vi "AdaptToInputs.vi"(3 "Term Types":T1[](array[typedef]), 4 "XRef":refnum<vi>, 5 "State In":T4={"Input Type"=variant(path path ""), "Terminals"=[]}) -> (0 "Reply":string[](array[string]), 2 "State Out":T4={"Input Type"=variant(path path ""), "Terminals"=[]})   [LabVIEW 2015, in "Await.xnode"]
doc: "This ability VI is called by LabVIEW during type propagation so that your XNode may adapt itself to new input types. Term Types is an array of pairs of current Term IDs and the type descriptors corresponding to them. The type descriptors are taken from the signal connected to the terminal. Unwired terminals are not included in the array. Use Reply to inform LabVIEW of any actions it needs to take.\n\nDefault behavior: None.\n\nThis ability does not provide UI and OS messages are not handled."
uses:
  Await.xnode
  State.ctl
  <vilib>/XNodeSupport/XNodeTermTypeIDPair.ctl
  <vilib>/XNodeSupport/XNodeType.ctl
  <vilib>/XNodeSupport/XNodeString.ctl
  <vilib>/Erdos Miller/LV-Scripting/LV-Scripting.lvlib
  <vilib>/Utility/Data Type/NI_Data Type.lvlib
  <vilib>/XNodeSupport/NI_XNodeSupport.lvlib
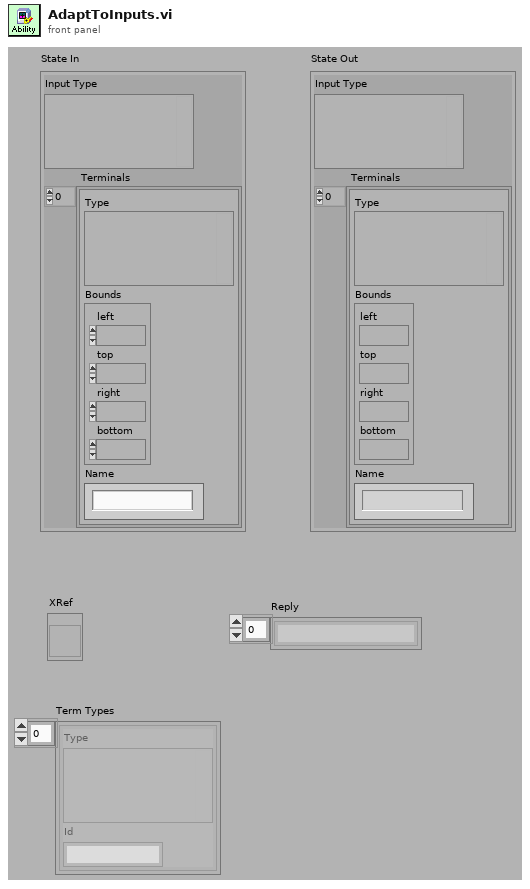
[diagram p1: front panel]
types:
  T1 = typedef "NI_XNodeSupport.lvlib/XNodeTermTypeIDPair.ctl" = cluster{"Type":T2, "Id":T3}
  T2 = typedef "NI_XNodeSupport.lvlib/XNodeType.ctl" = variant
  T3 = typedef "NI_XNodeSupport.lvlib/XNodeString.ctl" = string
  T4 = typedef "Await.xnode/State.ctl" = cluster{"Input Type":variant, "Terminals":cluster{"Type":variant, "Bounds":cluster{"left":i16, "top":i16, "right":i16, "bottom":i16}, "Name":string}[]}
  T5 = cluster{"Connector":i32, "Rects":cluster{"left":i16, "top":i16, "right":i16, "bottom":i16}[]}[]
  T6 = typedef "NI_Data Type.lvlib/VI Info.ctl" = cluster{"Connector Pane Pattern":i16, "Connector Pane Rotation":i16, "Flags":u32[], "Modification Date":timestamp, "Asynchronous":bool, "Non-Function":bool, "Subroutine":bool, "SubSystem":bool}
  T7 = cluster{"Connector":i32, "Rects":cluster{"left":i16, "top":i16, "right":i16, "bottom":i16}[]}
  T8 = cluster{"left":i16, "top":i16, "right":i16, "bottom":i16}[]
  T9 = cluster{"Variant":variant, "Rect":cluster{"left":i16, "top":i16, "right":i16, "bottom":i16}, "Name":string}
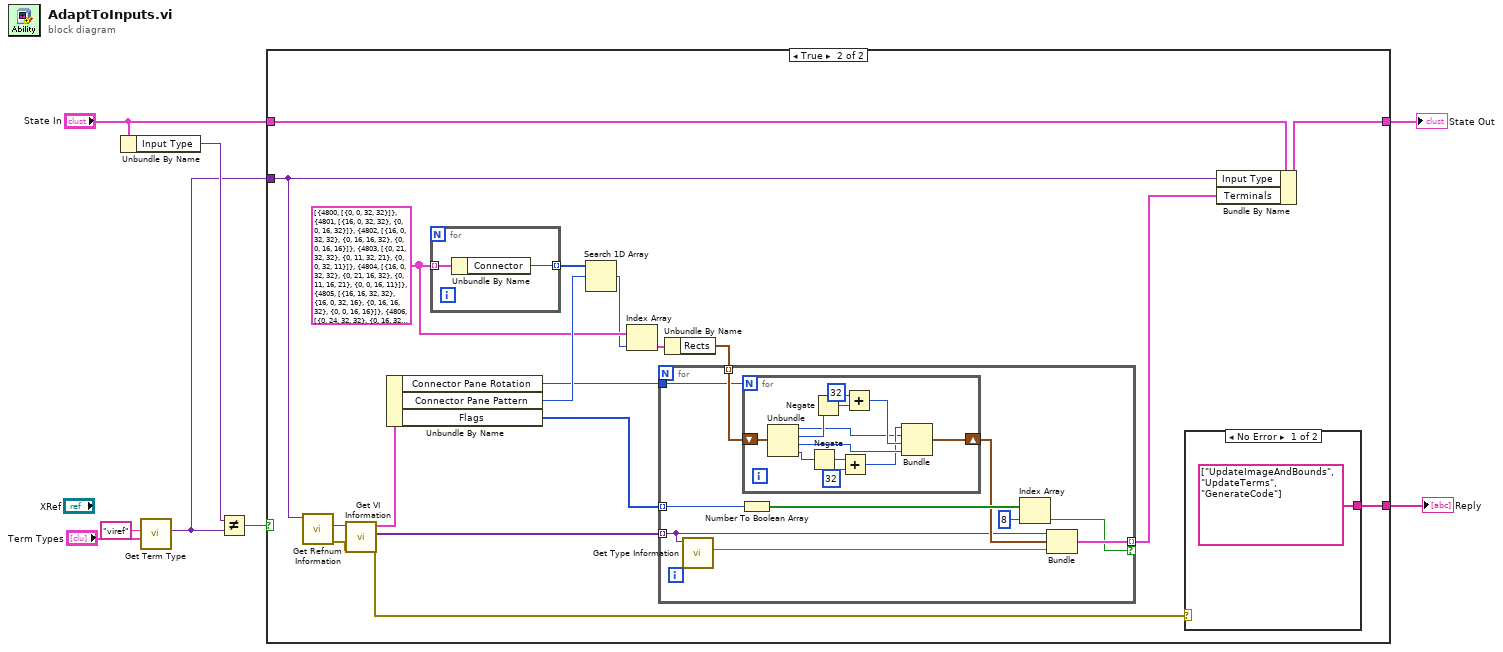
[diagram p0: block diagram]
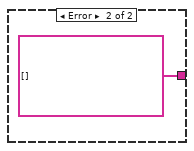
[diagram p3: hidden frame]
diagram:
  n1 = Unbundle By Name("State In") -> ("Input Type"=w6:variant)
  n2 = call <vilib>:"Get Term Type.vi"("Term Types"="Term Types", "ID"="viref") -> ("Type"=w2:variant)  [unwired: 9 in]
  n3 = Not Equal?(x=w6, y=w2) -> (x != y?=w5:bool)
  n4 = case shown="True" w5 {
    tunnel: [w9 w26] -> w4
    tunnel: "State In" -> [w9 w27]
    tunnel: w2 -> [_ w25]
    tunnel: [_ w13] -> w1
    frame False {
    }
    frame True {
      w18 = T5 [{"Connector"=4800, "Rects"=[{"left"=0, "top"=0, "right"=32, "bottom"=32}]}, {"Connector"=4801, "Rects"=[{"left"=16, "top"=0, "right"=32, "bottom"=32}, {"left"=0, "top"=0, "right"=16, "bottom"=32}]}, {"Connector"=4802, "Rects"=[{"left"=16, "top"=0, "right"=32, "bottom"=32}, {"left"=0, "top"=16, "right"=16, "bottom"=32}, {"left"=0, "top"=0, "right"=16, "bottom"=16}]}, {"Connector"=4803, "Rects"=[{"left"=0, "top"=21, "right"=32, "bottom"=32}, {"left"=0, "top"=11, "right"=32, "bottom"=21}, {"left"=0, "top"=0, "right"=32, "bottom"=11}]}, {"Connector"=4804, "Rects"=[{"left"=16, "top"=0, "right"=32, "bottom"=32}, {"left"=0, "top"=21, "right"=16, "bottom"=32}, {"left"=0, "top"=11, "right"=16, "bottom"=21}, {"left"=0, "top"=0, "right"=16, "bottom"=11}]}, {"Connector"=4805, "Rects"=[{"left"=16, "top"=16, "right"=32, "bottom"=32}, {"left"=16, "top"=0, "right"=32, "bottom"=16}, {"left"=0, "top"=16, "right"=16, "bottom"=32}, {"left"=0, "top"=0, "right"=16, "bottom"=16}]}, {"Connector"=4806, "Rects"=[{"left"=0, "top"=24, "right"=32, "bottom"=32}, {"left"=0, "top"=16, "right"=32, "bottom"=24}, {"left"=0, "top"=8, "right"=32, "bottom"=16}, {"left"=0, "top"=0, "right"=32, "bottom"=8}]}, {"Connector"=4807, "Rects"=[{"left"=16, "top"=16, "right"=32, "bottom"=32}, {"left"=16, "top"=0, "right"=32, "bottom"=16}, {"left"=0, "top"=21, "right"=16, "bottom"=32}, {"left"=0, "top"=11, "right"=16, "bottom"=21}, {"left"=0, "top"=0, "right"=16, "bottom"=11}]}, {"Connector"=4808, "Rects"=[{"left"=16, "top"=0, "right"=32, "bottom"=32}, {"left"=0, "top"=24, "right"=16, "bottom"=32}, {"left"=0, "top"=16, "right"=16, "bottom"=24}, {"left"=0, "top"=8, "right"=16, "bottom"=16}, {"left"=0, "top"=0, "right"=16, "bottom"=8}]}, {"Connector"=4809, "Rects"=[{"left"=16, "top"=16, "right"=32, "bottom"=32}, {"left"=16, "top"=0, "right"=32, "bottom"=16}, {"left"=0, "top"=24, "right"=16, "bottom"=32}, {"left"=0, "top"=16, "right"=16, "bottom"=24}, {"left"=0, "top"=8, "right"=16, "bottom"=16}, {"left"=0, "top"=0, "right"=16, "bottom"=8}]}, {"Connector"=4810, "Rects"=[{"left"=16, "top"=21, "right"=32, "bottom"=32}, {"left"=16, "top"=11, "right"=32, "bottom"=21}, {"left"=16, "top"=0, "right"=32, "bottom"=11}, {"left"=0, "top"=21, "right"=16, "bottom"=32}, {"left"=0, "top"=11, "right"=16, "bottom"=21}, {"left"=0, "top"=0, "right"=16, "bottom"=11}]}, {"Connector"=4811, "Rects"=[{"left"=16, "top"=21, "right"=32, "bottom"=32}, {"left"=16, "top"=11, "right"=32, "bottom"=21}, {"left"=16, "top"=0, "right"=32, "bottom"=11}, {"left"=0, "top"=24, "right"=16, "bottom"=32}, {"left"=0, "top"=16, "right"=16, "bottom"=24}, {"left"=0, "top"=8, "right"=16, "bottom"=16}, {"left"=0, "top"=0, "right"=16, "bottom"=8}]}, {"Connector"=4812, "Rects"=[{"left"=16, "top"=24, "right"=32, "bottom"=32}, {"left"=16, "top"=16, "right"=32, "bottom"=24}, {"left"=16, "top"=8, "right"=32, "bottom"=16}, {"left"=16, "top"=0, "right"=32, "bottom"=8}, {"left"=0, "top"=24, "right"=16, "bottom"=32}, {"left"=0, "top"=16, "right"=16, "bottom"=24}, {"left"=0, "top"=8, "right"=16, "bottom"=16}, {"left"=0, "top"=0, "right"=16, "bottom"=8}]}, {"Connector"=4813, "Rects"=[{"left"=16, "top"=24, "right"=32, "bottom"=32}, {"left"=16, "top"=16, "right"=32, "bottom"=24}, {"left"=16, "top"=8, "right"=32, "bottom"=16}, {"left"=16, "top"=0, "right"=32, "bottom"=8}, {"left"=8, "top"=0, "right"=16, "bottom"=32}, {"left"=0, "top"=24, "right"=8, "bottom"=32}, {"left"=0, "top"=16, "right"=8, "bottom"=24}, {"left"=0, "top"=8, "right"=8, "bottom"=16}, {"left"=0, "top"=0, "right"=8, "bottom"=8}]}, {"Connector"=4814, "Rects"=[{"left"=16, "top"=24, "right"=32, "bottom"=32}, {"left"=16, "top"=16, "right"=32, "bottom"=24}, {"left"=16, "top"=8, "right"=32, "bottom"=16}, {"left"=16, "top"=0, "right"=32, "bottom"=8}, {"left"=8, "top"=16, "right"=16, "bottom"=32}, {"left"=8, "top"=0, "right"=16, "bottom"=16}, {"left"=0, "top"=24, "right"=8, "bottom"=32}, {"left"=0, "top"=16, "right"=8, "bottom"=24}, {"left"=0, "top"=8, "right"=8, "bottom"=16}, {"left"=0, "top"=0, "right"=8, "bottom"=8}]}, {"Connector"=4815, "Rects"=[{"left"=24, "top"=24, "right"=32, "bottom"=32}, {"left"=24, "top"=16, "right"=32, "bottom"=24}, {"left"=24, "top"=8, "right"=32, "bottom"=16}, {"left"=24, "top"=0, "right"=32, "bottom"=8}, {"left"=16, "top"=16, "right"=24, "bottom"=32}, {"left"=16, "top"=0, "right"=24, "bottom"=16}, {"left"=8, "top"=16, "right"=16, "bottom"=32}, {"left"=8, "top"=0, "right"=16, "bottom"=16}, {"left"=0, "top"=24, "right"=8, "bottom"=32}, {"left"=0, "top"=16, "right"=8, "bottom"=24}, {"left"=0, "top"=8, "right"=8, "bottom"=16}, {"left"=0, "top"=0, "right"=8, "bottom"=8}]}, {"Connector"=4816, "Rects"=[{"left"=0, "top"=0, "right"=8, "bottom"=11}, {"left"=8, "top"=0, "right"=16, "bottom"=11}, {"left"=0, "top"=11, "right"=16, "bottom"=21}, {"left"=0, "top"=21, "right"=8, "bottom"=32}, {"left"=8, "top"=21, "right"=16, "bottom"=32}, {"left"=16, "top"=0, "right"=32, "bottom"=32}]}, {"Connector"=4817, "Rects"=[{"left"=0, "top"=0, "right"=8, "bottom"=11}, {"left"=8, "top"=0, "right"=16, "bottom"=11}, {"left"=0, "top"=11, "right"=16, "bottom"=21}, {"left"=0, "top"=21, "right"=8, "bottom"=32}, {"left"=8, "top"=21, "right"=16, "bottom"=32}, {"left"=16, "top"=0, "right"=32, "bottom"=16}, {"left"=16, "top"=16, "right"=32, "bottom"=32}]}, {"Connector"=4818, "Rects"=[{"left"=0, "top"=0, "right"=8, "bottom"=11}, {"left"=8, "top"=0, "right"=16, "bottom"=11}, {"left"=0, "top"=11, "right"=16, "bottom"=21}, {"left"=0, "top"=21, "right"=8, "bottom"=32}, {"left"=8, "top"=21, "right"=16, "bottom"=32}, {"left"=16, "top"=0, "right"=32, "bottom"=11}, {"left"=16, "top"=11, "right"=32, "bottom"=21}, {"left"=16, "top"=21, "right"=32, "bottom"=32}]}, {"Connector"=4819, "Rects"=[{"left"=0, "top"=0, "right"=8, "bottom"=11}, {"left"=8, "top"=0, "right"=16, "bottom"=11}, {"left"=0, "top"=11, "right"=16, "bottom"=21}, {"left"=0, "top"=21, "right"=8, "bottom"=32}, {"left"=8, "top"=21, "right"=16, "bottom"=32}, {"left"=16, "top"=0, "right"=32, "bottom"=8}, {"left"=16, "top"=8, "right"=32, "bottom"=16}, {"left"=16, "top"=16, "right"=32, "bottom"=24}, {"left"=16, "top"=24, "right"=32, "bottom"=32}]}, {"Connector"=4820, "Rects"=[{"left"=0, "top"=0, "right"=8, "bottom"=11}, {"left"=8, "top"=0, "right"=16, "bottom"=11}, {"left"=0, "top"=11, "right"=16, "bottom"=21}, {"left"=0, "top"=21, "right"=8, "bottom"=32}, {"left"=8, "top"=21, "right"=16, "bottom"=32}, {"left"=16, "top"=0, "right"=24, "bottom"=11}, {"left"=24, "top"=0, "right"=32, "bottom"=11}, {"left"=16, "top"=11, "right"=32, "bottom"=21}, {"left"=16, "top"=21, "right"=24, "bottom"=32}, {"left"=24, "top"=21, "right"=32, "bottom"=32}]}, {"Connector"=4821, "Rects"=[{"left"=0, "top"=0, "right"=8, "bottom"=11}, {"left"=8, "top"=0, "right"=16, "bottom"=11}, {"left"=0, "top"=11, "right"=16, "bottom"=21}, {"left"=0, "top"=21, "right"=8, "bottom"=32}, {"left"=8, "top"=21, "right"=16, "bottom"=32}, {"left"=16, "top"=0, "right"=24, "bottom"=16}, {"left"=24, "top"=0, "right"=32, "bottom"=8}, {"left"=24, "top"=8, "right"=32, "bottom"=16}, {"left"=16, "top"=16, "right"=24, "bottom"=32}, {"left"=24, "top"=16, "right"=32, "bottom"=24}, {"left"=24, "top"=24, "right"=32, "bottom"=32}]}, {"Connector"=4822, "Rects"=[{"left"=0, "top"=0, "right"=8, "bottom"=8}, {"left"=8, "top"=0, "right"=16, "bottom"=16}, {"left"=0, "top"=8, "right"=8, "bottom"=16}, {"left"=0, "top"=16, "right"=8, "bottom"=24}, {"left"=8, "top"=16, "right"=16, "bottom"=32}, {"left"=0, "top"=24, "right"=8, "bottom"=32}, {"left"=16, "top"=0, "right"=32, "bottom"=11}, {"left"=16, "top"=11, "right"=32, "bottom"=21}, {"left"=16, "top"=21, "right"=32, "bottom"=32}]}, {"Connector"=4823, "Rects"=[{"left"=0, "top"=0, "right"=8, "bottom"=8}, {"left"=0, "top"=8, "right"=8, "bottom"=16}, {"left"=0, "top"=16, "right"=8, "bottom"=24}, {"left"=0, "top"=24, "right"=8, "bottom"=32}, {"left"=8, "top"=0, "right"=16, "bottom"=32}, {"left"=16, "top"=0, "right"=32, "bottom"=32}]}, {"Connector"=4824, "Rects"=[{"left"=0, "top"=0, "right"=8, "bottom"=8}, {"left"=0, "top"=8, "right"=8, "bottom"=16}, {"left"=0, "top"=16, "right"=8, "bottom"=24}, {"left"=0, "top"=24, "right"=8, "bottom"=32}, {"left"=8, "top"=0, "right"=16, "bottom"=32}, {"left"=16, "top"=0, "right"=32, "bottom"=16}, {"left"=16, "top"=16, "right"=32, "bottom"=32}]}, {"Connector"=4825, "Rects"=[{"left"=0, "top"=0, "right"=8, "bottom"=8}, {"left"=0, "top"=8, "right"=8, "bottom"=16}, {"left"=0, "top"=16, "right"=8, "bottom"=24}, {"left"=0, "top"=24, "right"=8, "bottom"=32}, {"left"=8, "top"=0, "right"=16, "bottom"=32}, {"left"=16, "top"=0, "right"=32, "bottom"=11}, {"left"=16, "top"=11, "right"=32, "bottom"=21}, {"left"=16, "top"=21, "right"=32, "bottom"=32}]}, {"Connector"=4826, "Rects"=[{"left"=24, "top"=24, "right"=32, "bottom"=32}, {"left"=24, "top"=16, "right"=32, "bottom"=24}, {"left"=24, "top"=8, "right"=32, "bottom"=16}, {"left"=24, "top"=0, "right"=32, "bottom"=8}, {"left"=16, "top"=0, "right"=24, "bottom"=32}, {"left"=8, "top"=0, "right"=16, "bottom"=32}, {"left"=0, "top"=24, "right"=8, "bottom"=32}, {"left"=0, "top"=16, "right"=8, "bottom"=24}, {"left"=0, "top"=8, "right"=8, "bottom"=16}, {"left"=0, "top"=0, "right"=8, "bottom"=8}]}, {"Connector"=4827, "Rects"=[{"left"=16, "top"=0, "right"=32, "bottom"=32}, {"left"=8, "top"=16, "right"=16, "bottom"=32}, {"left"=8, "top"=0, "right"=16, "bottom"=16}, {"left"=0, "top"=24, "right"=8, "bottom"=32}, {"left"=0, "top"=16, "right"=8, "bottom"=24}, {"left"=0, "top"=8, "right"=8, "bottom"=16}, {"left"=0, "top"=0, "right"=8, "bottom"=8}]}, {"Connector"=4828, "Rects"=[{"left"=16, "top"=16, "right"=32, "bottom"=32}, {"left"=16, "top"=0, "right"=32, "bottom"=16}, {"left"=8, "top"=16, "right"=16, "bottom"=32}, {"left"=8, "top"=0, "right"=16, "bottom"=16}, {"left"=0, "top"=24, "right"=8, "bottom"=32}, {"left"=0, "top"=16, "right"=8, "bottom"=24}, {"left"=0, "top"=8, "right"=8, "bottom"=16}, {"left"=0, "top"=0, "right"=8, "bottom"=8}]}, {"Connector"=4829, "Rects"=[{"left"=24, "top"=24, "right"=32, "bottom"=32}, {"left"=24, "top"=16, "right"=32, "bottom"=24}, {"left"=24, "top"=8, "right"=32, "bottom"=16}, {"left"=24, "top"=0, "right"=32, "bottom"=8}, {"left"=16, "top"=0, "right"=24, "bottom"=32}, {"left"=8, "top"=16, "right"=16, "bottom"=32}, {"left"=8, "top"=0, "right"=16, "bottom"=16}, {"left"=0, "top"=24, "right"=8, "bottom"=32}, {"left"=0, "top"=16, "right"=8, "bottom"=24}, {"left"=0, "top"=8, "right"=8, "bottom"=16}, {"left"=0, "top"=0, "right"=8, "bottom"=8}]}, {"Connector"=4830, "Rects"=[{"left"=21, "top"=0, "right"=32, "bottom"=32}, {"left"=11, "top"=0, "right"=21, "bottom"=32}, {"left"=0, "top"=16, "right"=11, "bottom"=32}, {"left"=0, "top"=0, "right"=11, "bottom"=16}]}, {"Connector"=4831, "Rects"=[{"left"=21, "top"=0, "right"=32, "bottom"=32}, {"left"=11, "top"=0, "right"=21, "bottom"=32}, {"left"=0, "top"=21, "right"=11, "bottom"=32}, {"left"=0, "top"=11, "right"=11, "bottom"=21}, {"left"=0, "top"=0, "right"=11, "bottom"=11}]}, {"Connector"=4832, "Rects"=[{"left"=21, "top"=16, "right"=32, "bottom"=32}, {"left"=21, "top"=0, "right"=32, "bottom"=16}, {"left"=11, "top"=0, "right"=21, "bottom"=32}, {"left"=0, "top"=21, "right"=11, "bottom"=32}, {"left"=0, "top"=11, "right"=11, "bottom"=21}, {"left"=0, "top"=0, "right"=11, "bottom"=11}]}, {"Connector"=4833, "Rects"=[{"left"=0, "top"=0, "right"=7, "bottom"=7}, {"left"=7, "top"=0, "right"=13, "bottom"=16}, {"left"=13, "top"=0, "right"=19, "bottom"=16}, {"left"=19, "top"=0, "right"=25, "bottom"=16}, {"left"=25, "top"=0, "right"=32, "bottom"=7}, {"left"=0, "top"=7, "right"=7, "bottom"=13}, {"left"=25, "top"=7, "right"=32, "bottom"=13}, {"left"=0, "top"=13, "right"=7, "bottom"=19}, {"left"=25, "top"=13, "right"=32, "bottom"=19}, {"left"=0, "top"=19, "right"=7, "bottom"=25}, {"left"=25, "top"=19, "right"=32, "bottom"=25}, {"left"=0, "top"=25, "right"=7, "bottom"=32}, {"left"=7, "top"=16, "right"=13, "bottom"=32}, {"left"=13, "top"=16, "right"=19, "bottom"=32}, {"left"=19, "top"=16, "right"=25, "bottom"=32}, {"left"=25, "top"=25, "right"=32, "bottom"=32}]}, {"Connector"=4834, "Rects"=[{"left"=0, "top"=0, "right"=6, "bottom"=6}, {"left"=0, "top"=6, "right"=6, "bottom"=11}, {"left"=0, "top"=11, "right"=6, "bottom"=16}, {"left"=0, "top"=16, "right"=6, "bottom"=21}, {"left"=0, "top"=21, "right"=6, "bottom"=26}, {"left"=0, "top"=26, "right"=6, "bottom"=32}, {"left"=6, "top"=0, "right"=11, "bottom"=16}, {"left"=6, "top"=16, "right"=11, "bottom"=32}, {"left"=11, "top"=0, "right"=16, "bottom"=16}, {"left"=11, "top"=16, "right"=16, "bottom"=32}, {"left"=16, "top"=0, "right"=21, "bottom"=16}, {"left"=16, "top"=16, "right"=21, "bottom"=32}, {"left"=21, "top"=0, "right"=26, "bottom"=16}, {"left"=21, "top"=16, "right"=26, "bottom"=32}, {"left"=26, "top"=0, "right"=32, "bottom"=6}, {"left"=26, "top"=6, "right"=32, "bottom"=11}, {"left"=26, "top"=11, "right"=32, "bottom"=16}, {"left"=26, "top"=16, "right"=32, "bottom"=21}, {"left"=26, "top"=21, "right"=32, "bottom"=26}, {"left"=26, "top"=26, "right"=32, "bottom"=32}]}, {"Connector"=4835, "Rects"=[{"left"=0, "top"=0, "right"=4, "bottom"=4}, {"left"=0, "top"=4, "right"=4, "bottom"=8}, {"left"=0, "top"=8, "right"=4, "bottom"=12}, {"left"=0, "top"=12, "right"=4, "bottom"=16}, {"left"=0, "top"=16, "right"=4, "bottom"=20}, {"left"=0, "top"=20, "right"=4, "bottom"=24}, {"left"=0, "top"=24, "right"=4, "bottom"=28}, {"left"=0, "top"=28, "right"=4, "bottom"=32}, {"left"=4, "top"=0, "right"=8, "bottom"=16}, {"left"=4, "top"=16, "right"=8, "bottom"=32}, {"left"=8, "top"=0, "right"=12, "bottom"=16}, {"left"=8, "top"=16, "right"=12, "bottom"=32}, {"left"=12, "top"=0, "right"=16, "bottom"=16}, {"left"=12, "top"=16, "right"=16, "bottom"=32}, {"left"=16, "top"=0, "right"=20, "bottom"=16}, {"left"=16, "top"=16, "right"=20, "bottom"=32}, {"left"=20, "top"=0, "right"=24, "bottom"=16}, {"left"=20, "top"=16, "right"=24, "bottom"=32}, {"left"=24, "top"=0, "right"=28, "bottom"=16}, {"left"=24, "top"=16, "right"=28, "bottom"=32}, {"left"=28, "top"=0, "right"=32, "bottom"=4}, {"left"=28, "top"=4, "right"=32, "bottom"=8}, {"left"=28, "top"=8, "right"=32, "bottom"=12}, {"left"=28, "top"=12, "right"=32, "bottom"=16}, {"left"=28, "top"=16, "right"=32, "bottom"=20}, {"left"=28, "top"=20, "right"=32, "bottom"=24}, {"left"=28, "top"=24, "right"=32, "bottom"=28}, {"left"=28, "top"=28, "right"=32, "bottom"=32}]}] ("Array")
      n5 = call <vilib>:"Get Refnum Information.vi"("Variant"=w25) -> ("error out"=w12:errorcluster, "Strict Type"=w24:variant)  [unwired: 7 in, 2 out]
      n6 = call <vilib>:"Get VI Information.vi"("error in (no error)"=w12, "Variant"=w24) -> ("error out"=w11:errorcluster, "VI Terminal Types"=w21:variant[], "VI Info"=w23:T6)  [unwired: 6 in, 1 out]
      n7 = Unbundle By Name(w23) -> ("Connector Pane Rotation"=w10:i16, "Connector Pane Pattern"=w19:i16, "Flags"=w22:u32[])
      n8 = for {
        tunnel: w18 -> [w31] mode=indexing
        tunnel: [w30] -> w20 mode=indexing
        n9 = Unbundle By Name(w31) -> ("Connector"=w30:i32)
      }
      n10 = Search 1D Array(1D array=w20, element=w19) -> (index of element=w17:i32)  [unwired: 1 in]
      n11 = Index Array(array=w18, index=w17) -> (element=w16:T7)
      n12 = Unbundle By Name(w16) -> ("Rects"=w15:T8)
      n13 = for {
        tunnel: w22 -> [w41] mode=indexing
        tunnel: w21 -> [w32] mode=indexing
        tunnel: [w38] -> w14 mode=indexing if=w37
        tunnel: w15 -> [w35] mode=indexing
        tunnel: w10 -> [w33]
        n14 = call <vilib>:"Get Type Information.vi"("Variant"=w32) -> ("Name"=w36:string)  [unwired: 6 in, 4 out]
        n15 = Number To Boolean Array(number=w41) -> (Boolean array=w40:bool[])
        n16 = for {
          N: w33 -> [_]
          shift-right: [w44] -> w34
          shift-left: w35 -> [w53]
          n17 = Unbundle(w53) -> ("left"=w42:i16, "top"=w52:i16, "right"=w48:i16, "bottom"=w45:i16)
          n18 = Negate(x=w45) -> (-x=w46:i16)
          n19 = Negate(x=w52) -> (-x=w51:i16)
          n20 = Add(x=w46, y=i16 32 ("x")) -> (x+y=w43:i16)
          n21 = Add(x=i16 32, y=w51) -> (x+y=w49:i16)
          n22 = Bundle(w43, "left"=w42, w49, "right"=w48) -> (w44:cluster{i16, "left":i16, i16, "right":i16})  [unwired: 1 in]
        }
        n23 = Index Array(array=w40, index=8) -> (element=w37:bool)
        n24 = Bundle("Variant"=w32, "Rect"=w34, "Name"=w36) -> (w38:T9)  [unwired: 1 in]
      }
      n25 = case shown="No Error" w11 {
        tunnel: [string[] ["UpdateImageAndBounds", "UpdateTerms", "GenerateCode"] ("Reply") string[] [] ("Reply")] -> w13
        frame No Error {
        }
        frame Error {
        }
      }
      n26 = Bundle By Name(cluster=w27, "Input Type"=w25, "Terminals"=w14) -> (w26:T4)
    }
  }
  "Reply" <- w1
  "State Out" <- w4
